vi "Set_Cluster_Argument.vi"(1 "Clust Refnum":refnum<vi>, 2 "Prefix":string, 3 "Argument List In":string[](array[string])) -> (0 "Argument List Out":string[](array[string]))   [LabVIEW 2011]
doc: "This VI parses an argument to find it's text value. For example, given an argument in the form of Arg(\"some text\"), it would return \"some text\", without quotation marks."
uses:
  high_level_proc/source_dilution.ctl
  high_level_proc/source_noDilution.ctl
panel:
  out "error out":errorcluster
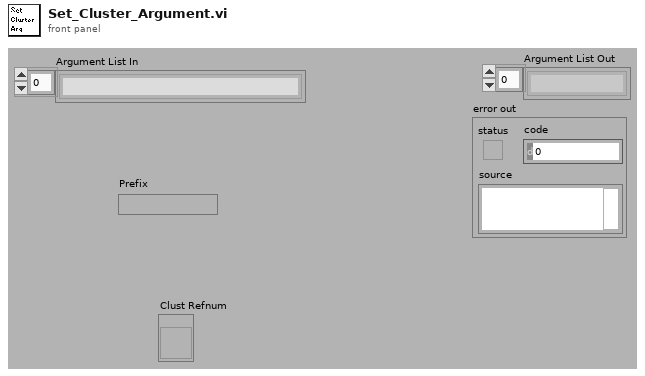
[diagram p1: front panel]
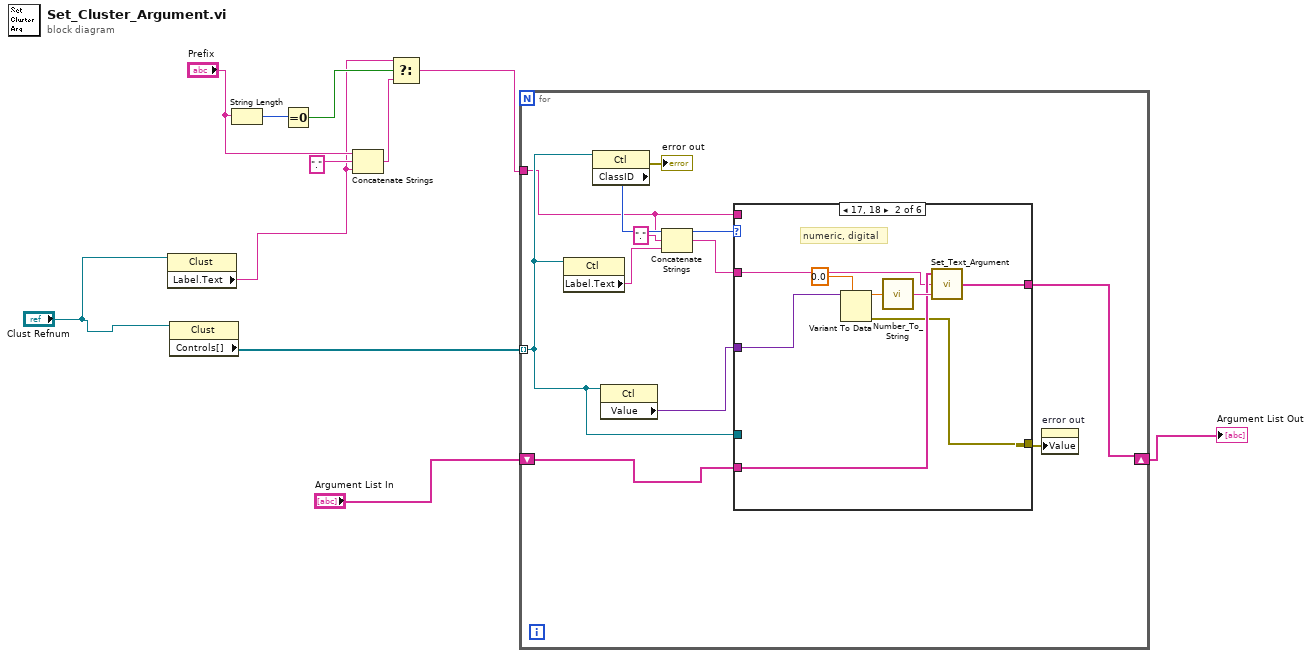
[diagram p0: block diagram]
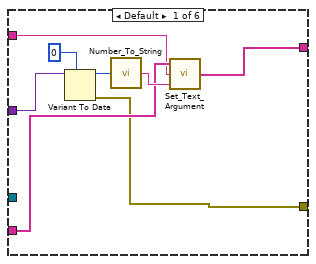
[diagram p2: hidden frame]
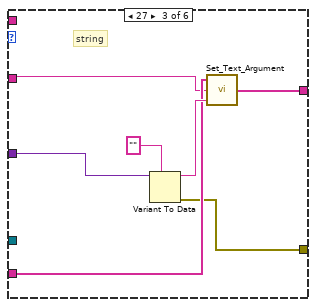
[diagram p3: hidden frame]
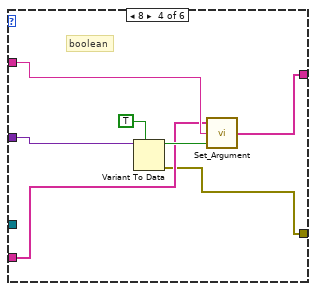
[diagram p4: hidden frame]
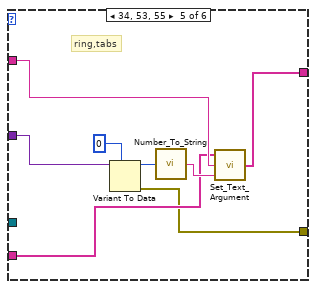
[diagram p5: hidden frame]
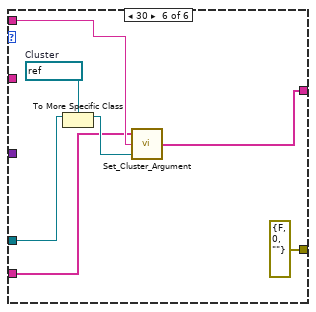
[diagram p6: hidden frame]
diagram:
  n1 = property class="Clust"(reference="Clust Refnum") -> ("Label.Text"=w2:string)  [unwired: 1 in, 2 out]
  n2 = property class="Clust"(reference="Clust Refnum") -> ("Controls[]"=w9:refnum<vi>[])  [unwired: 1 in, 2 out]
  n3 = String Length(string="Prefix") -> (length=w7:i32)
  n4 = Equal To 0?(x=w7) -> (x = 0?=w6:bool)
  n5 = Concatenate Strings("Prefix", "." ("string"), w2) -> (w4:string)
  n6 = Select(t=w2, s=w6, f=w4) -> (s? t:f=w1:string)
  n7 = for {
    tunnel: w9 -> [w13] mode=indexing
    shift-right: [w20] -> w10
    shift-left: "Argument List In" -> [w21]
    tunnel: w1 -> [w12]
    n8 = property class="Ctl"(reference=w13) -> ("Label.Text"=w16:string)  [unwired: 1 in, 2 out]
    n9 = property class="Ctl"(reference=w13) -> (error out=→"error out":errorcluster, "ClassID"=w22:u32)  [unwired: 1 in, 1 out]
    n10 = property class="Ctl"(reference=w13) -> ("Value"=w19:variant)  [unwired: 1 in, 2 out]
    n11 = Concatenate Strings(w12, "." ("string"), w16) -> (w14:string)
    n12 = case shown="17, 18" w22 {
      tunnel: w21 -> [w27 w35 w44 w49 w55 w63]
      tunnel: [w23 w34 w41 w47 w53 w61] -> w20
      tunnel: w14 -> [w26 w33 w43 w50 w56 _]
      tunnel: w19 -> [w25 w32 w40 w46 w57 _]
      tunnel: [w24 w31 w42 w48 w54 errorcluster {"status"=FALSE, "code"=0, "source"=""} ("error out")] -> w17
      tunnel: w13 -> [_ _ _ _ _ w67]
      tunnel: w12 -> [_ _ _ _ _ w64]
      frame Default {
        n13 = Variant To Data(type=0, Variant=w25) -> (data=w28:i32, error out=w24:errorcluster)  [unwired: 1 in]
        n14 = call "Number_To_String.vi"("Number"=w28) -> ("String"=w30:string)
        n15 = call "Set_Text_Argument.vi"("Text"=w30, "Argument"=w26, "Argument List In"=w27) -> ("Argument List Out"=w23:string[])
      }
      frame 17, 18 {
        # "numeric, digital"
        n16 = Variant To Data(type=0.0, Variant=w32) -> (data=w37:dbl, error out=w31:errorcluster)  [unwired: 1 in]
        n17 = call "Number_To_String.vi"("Number"=w37) -> ("String"=w36:string)
        n18 = call "Set_Text_Argument.vi"("Text"=w36, "Argument"=w33, "Argument List In"=w35) -> ("Argument List Out"=w34:string[])
      }
      frame 27 {
        # "string"
        n19 = Variant To Data(type="", Variant=w40) -> (data=w45:string, error out=w42:errorcluster)  [unwired: 1 in]
        n20 = call "Set_Text_Argument.vi"("Text"=w45, "Argument"=w43, "Argument List In"=w44) -> ("Argument List Out"=w41:string[])
      }
      frame 8 {
        # "boolean"
        n21 = Variant To Data(type=TRUE, Variant=w46) -> (data=w51:bool, error out=w48:errorcluster)  [unwired: 1 in]
        n22 = call "Set_Argument.vi"("Enable"=w51, "Argument"=w50, "Argument List In"=w49) -> ("Argument List Out"=w47:string[])
      }
      frame 34, 53, 55 {
        # "ring,tabs"
        n23 = Variant To Data(type=u16 0, Variant=w57) -> (data=w58:u16, error out=w54:errorcluster)  [unwired: 1 in]
        n24 = call "Number_To_String.vi"("Number"=w58) -> ("String"=w60:string)
        n25 = call "Set_Text_Argument.vi"("Text"=w60, "Argument"=w56, "Argument List In"=w55) -> ("Argument List Out"=w53:string[])
      }
      frame 30 {
        w66 = refnum<vi> refnum  # Cluster
        n26 = To More Specific Class(target class=w66, reference=w67) -> (specific class reference=w65:refnum<vi>)  [unwired: 1 in, 1 out]
        n27 = call "Set_Cluster_Argument.vi"("Clust Refnum"=w65, "Prefix"=w64, "Argument List In"=w63) -> ("Argument List Out"=w61:string[])
      }
    }
    n28 = property on="error out" class="Clust (strict)"("Value"=w17) -> ()  [unwired: 2 in, 2 out]
  }
  "Argument List Out" <- w10
